vi "Commit Calibration Data Dll.vi"(0 "CART TCP Connection In":refnum<k5>, 5 "CommitMemory":string="Commit Memory=eeprom") -> (4 "CART TCP Connection Out":refnum<k5>, 15 "StatusIsFalse":i16)   [LabVIEW 2011]
panel:
  out "TCP Messages":string[](array[string])
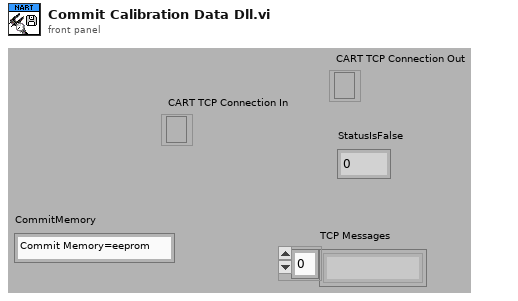
[diagram p1: front panel]
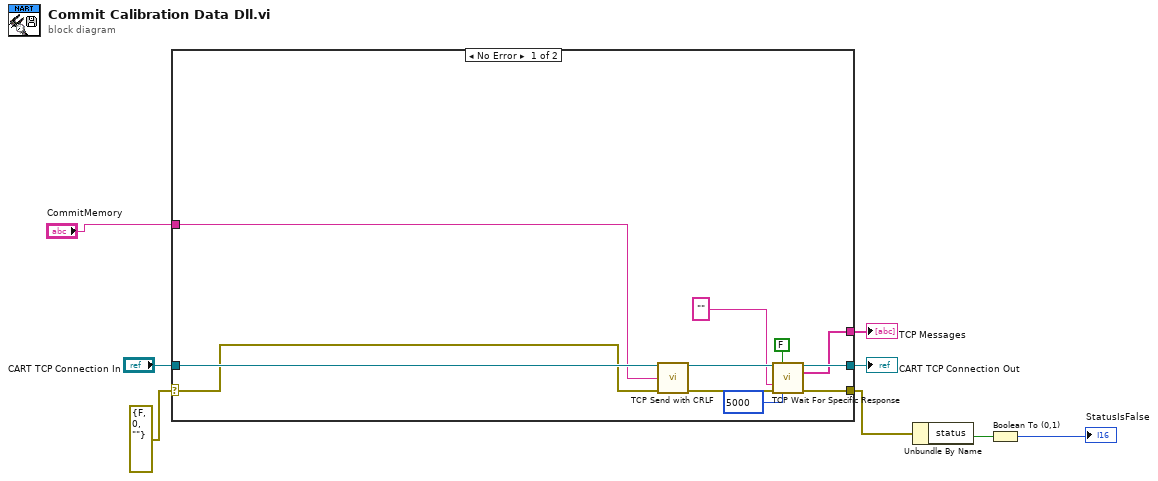
[diagram p0: block diagram]
diagram:
  n1 = case shown="No Error" errorcluster {"status"=FALSE, "code"=0, "source"=""} ("error in (no error)") {
    selector: errorcluster {"status"=FALSE, "code"=0, "source"=""} ("error in (no error)") -> [w18 w21]
    tunnel: [w15 w21] -> w4
    tunnel: "CART TCP Connection In" -> [w19 w20]
    tunnel: [w16 w20] -> w6
    tunnel: [w12 _] -> w5
    tunnel: "CommitMemory" -> [w9 _]
    frame No Error {
      n2 = call "TCP Send with CRLF.vi"("CART TCP Connection"=w19, "data in"=w9, "error IO"=w18) -> ("CART TCP Connection Out"=w17:refnum<k5>, "error out"=w14:errorcluster)  [unwired: 11 in]
      n3 = call "TCP Wait For Specific Response.vi"("TCP Connection In"=w17, "Next response (t)"=FALSE, "Expected Message Start (\"\":any)"="" ("Expected Message Start (\"\":any)"), "error in"=w14, "Timeout (250 ms)"=5000) -> ("TCP Connection Out"=w16:refnum<k5>, "TCP Messages"=w12:string[], "error out"=w15:errorcluster)  [unwired: 7 in, 1 out]
    }
    frame Error {
    }
  }
  "CART TCP Connection Out" <- w6
  "TCP Messages" <- w5
  n4 = Unbundle By Name(w4) -> ("status"=w3:bool)
  n5 = Boolean To (0,1)(Boolean=w3) -> (0, 1=→"StatusIsFalse":i16)
